vi "makeDecisions.vi"(8 "error in (no error)":errorcluster, 10 "model":refnum<class "Model.lvclass">, 11 "SoakingState in":refnum<class "SoakingState.lvclass">) -> (0 "error out":errorcluster, 2 "model 2":refnum<class "Model.lvclass">, 3 "SoakingState out":refnum<class "SoakingState.lvclass">)   [LabVIEW 2013, in "SoakingState.lvclass"]
uses:
  SoakingState.lvclass
  Model/Model/Model.lvclass
  ExecutingCycleState/ExecutingCycleState.lvclass
  Typedefs/StateSelector.ctl
  Typedefs/AITDTTypedefs.lvlib
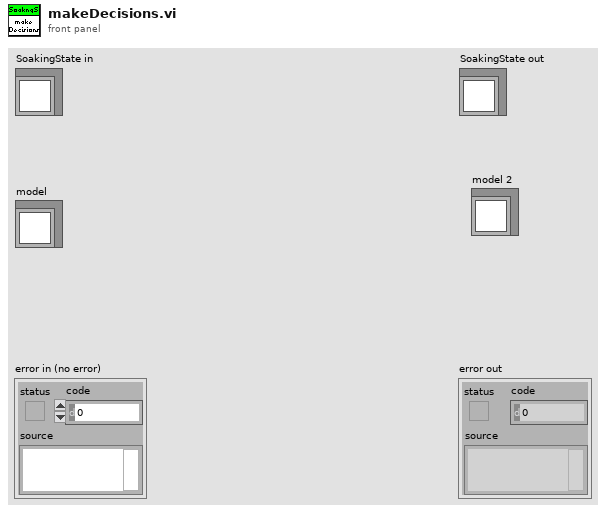
[diagram p1: front panel]
types:
  T1 = typedef "AITDTTypedefs.lvlib/StateSelector.ctl" = enum16{"AwaitingSetpointAcknowledgmentState", "EndingCycleState", "FaultState", "OffState", "PausingState", "RequestingNewSetpointState", "SamplingState", "SettlingState", "SoakingState", "StabilizingState", "StandbyState", "StoppedState", "TransitioningTemperatureState"}
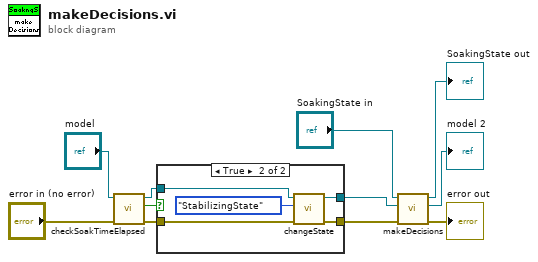
[diagram p0: block diagram]
diagram:
  n1 = call "checkSoakTimeElapsed.vi"("error in (no error)"="error in (no error)", "Model in"="model") -> ("error out"=w3:errorcluster, "soakTimeHasElapsedIsTrue"=w5:bool, "Model out"=w6:refnum<class "Model.lvclass">)  [unwired: 7 in]
  n2 = case shown="True" w5 {
    tunnel: w6 -> [w13 w15]
    tunnel: w3 -> [w12 w14]
    tunnel: [w12 w17] -> w1
    tunnel: [w13 w16] -> w2
    frame False {
    }
    frame True {
      n3 = call "changeState.vi"("error in (no error)"=w14, "State:"=StateSelector."StabilizingState", "Model in"=w15) -> ("error out"=w17:errorcluster, "Model out"=w16:refnum<class "Model.lvclass">)  [unwired: 7 in]
    }
  }
  n4 = call-parent "makeDecisions.vi"("error in (no error)"=w1, "model"=w2, "EnabledState in"="SoakingState in") -> ("error out"=→"error out":errorcluster, "model 2"=→"model 2":refnum<class "Model.lvclass">, "EnabledState out"=→"SoakingState out":refnum<class "SoakingState.lvclass">)  [unwired: 6 in]
